vi "RT.vi"() -> ()   [LabVIEW 2020]
uses:
  <vilib>/FPGAPlugInAG/cRIO-9054/niLvFpga_Open_cRIO-9054.vi
  <vilib>/FPGAPlugInAG/cRIO-9054/niLvFpga_Reset_cRIO-9054.vi
  <vilib>/Utility/error.llb/Error Cluster From Error Code.vi
  <vilib>/rvi/errors/niLvFpgaAdjustHostInterfaceError.vi
  <vilib>/FPGAPlugInAG/cRIO-9054/niLvFpga_Run_cRIO-9054.vi
  <vilib>/FPGAPlugInAG/cRIO-9054/niLvFpga_Close_cRIO-9054.vi
  <vilib>/rvi/interface/nirviOpenFPGA/nirviOpenFPGA.xnode
  FPGA Bitfiles/8192.lvbitx
  <vilib>/rvi/interface/nirviMethod/nirviMethod.xnode
  <vilib>/rvi/interface/nirviReadWriteControl/nirviReadWriteControl.xnode
  <vilib>/rvi/interface/nirviCloseFPGA/nirviCloseFPGA.xnode
  <vilib>/rvi/errors/niLvFpgaMergeErrorWithErrorCode.vi
  <vilib>/FPGAPlugInAG/cRIO-9054/niLvFpga_ReadFifo_cRIO-9054.vi
  NiFpgaLv.dll
  <vilib>/FPGAPlugInAG/cRIO-9054/niLvFpga_StartFifo_cRIO-9054.vi
panel:
  in  "FFT length":i32=8192
  out "Timing Chart":waveform(i16)(graph)
  in  "FFT loop iterations":i32
  in  "auto stop":bool=TRUE
  out "FFT time (uSec)":u32
  out "data collection time (uSec)":u32
  out "FFT Spectrum":waveform(dbl)(graph)
  out "Actual loop rate (Hz)":dbl
  out "aquired data":waveform(dbl)(graph)
  in  "number of date points":i32=9000
  out "Timed Out?":bool
  in  "requested Loop rate (Hz)":u32=1000
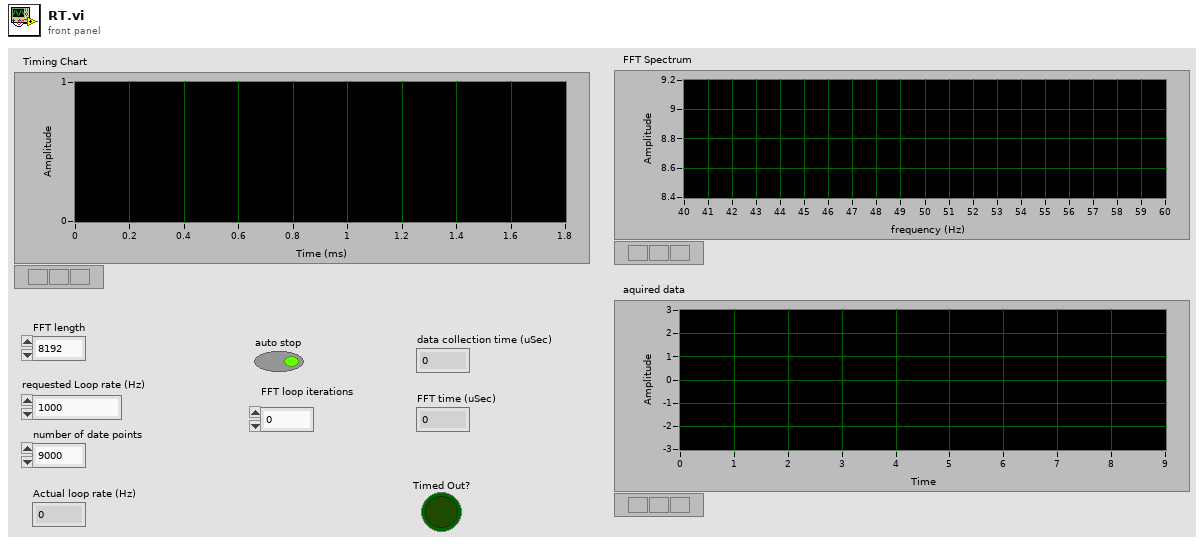
[diagram p1: front panel]
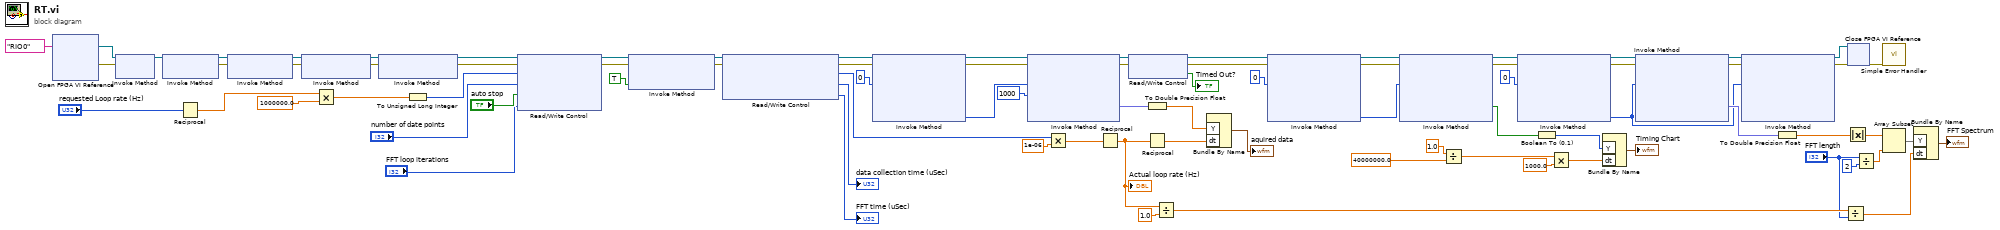
[diagram p0: block diagram]
diagram:
  n1 = xnode "Open FPGA VI Reference"("resource name"=tag "RIO0") -> ("FPGA VI Reference Out"=w33:refnum<k20>, "error out"=w32:errorcluster)  [unwired: 1 in]
  n2 = xnode "Invoke Method"("FPGA VI Reference In"=w33, "error in"=w32) -> ("FPGA VI Reference Out"=w11:refnum<k20>)  [unwired: 1 out]
  n3 = xnode "Invoke Method"("FPGA VI Reference In"=w11) -> ("FPGA VI Reference Out"=w10:refnum<k20>, "error out"=w9:errorcluster)  [unwired: 1 in]
  n4 = Reciprocal(x="requested Loop rate (Hz)") -> (1/x=w69:dbl)
  n5 = xnode "Invoke Method"("FPGA VI Reference In"=w10, "error in"=w9) -> ("FPGA VI Reference Out"=w15:refnum<k20>, "error out"=w14:errorcluster)
  n6 = xnode "Invoke Method"("FPGA VI Reference In"=w15, "error in"=w14) -> ("FPGA VI Reference Out"=w13:refnum<k20>, "error out"=w12:errorcluster)
  n7 = Multiply(x=w69, y=1000000.0) -> (x*y=w67:dbl)
  n8 = xnode "Invoke Method"("FPGA VI Reference In"=w13, "error in"=w12) -> ("FPGA VI Reference Out"=w18:refnum<k20>, "error out"=w17:errorcluster)
  n9 = To Unsigned Long Integer(number=w67) -> (unsigned 32bit integer=w66:u32)
  n10 = xnode "Read/Write Control"("FPGA VI Reference In"=w18, "error in"=w17, "Rate (uSec)"=w66, "Loop number"="number of date points", "auto stop"="auto stop", "FFT loop iterations"="FFT loop iterations") -> ("FPGA VI Reference Out"=w81:refnum<k20>, "error out"=w80:errorcluster)
  n11 = xnode "Invoke Method"("FPGA VI Reference In"=w81, "error in"=w80, "Wait Until Done (F)"=TRUE) -> ("FPGA VI Reference Out"=w77:refnum<k20>, "error out"=w76:errorcluster)
  n12 = xnode "Read/Write Control"("FPGA VI Reference In"=w77, "error in"=w76) -> ("FPGA VI Reference Out"=w30:refnum<k20>, "error out"=w29:errorcluster, "Actual loop rate"=w72:u32, "data collection time (uSec)"=→"data collection time (uSec)":u32, "FFT time (uSec)"=→"FFT time (uSec)":u32)
  n13 = xnode "Invoke Method"("FPGA VI Reference In"=w30, "error in"=w29, "Number of Elements"=u32 0) -> ("FPGA VI Reference Out"=w28:refnum<k20>, "error out"=w27:errorcluster, "Elements Remaining"=w25:u32)  [unwired: 1 in, 1 out]
  n14 = xnode "Invoke Method"("FPGA VI Reference In"=w28, "error in"=w27, "Number of Elements"=w25, "Timeout (ms)"=1000) -> ("FPGA VI Reference Out"=w75:refnum<k20>, "error out"=w74:errorcluster, "Data"=w39:fxp<+/-,24,7>[])  [unwired: 1 out]
  n15 = Multiply(x=w72, y=1e-06) -> (x*y=w70:dbl)
  n16 = Reciprocal(x=w70) -> (1/x=w35:dbl)
  "Actual loop rate (Hz)" <- w35
  n17 = xnode "Read/Write Control"("FPGA VI Reference In"=w75, "error in"=w74) -> ("FPGA VI Reference Out"=w46:refnum<k20>, "error out"=w45:errorcluster, "Timed Out?"=→"Timed Out?":bool)
  n18 = Reciprocal(x=w35) -> (1/x=w62:dbl)
  n19 = To Double Precision Float(number=w39) -> (double precision float=w63:dbl[])
  n20 = Divide(x=w35, y=1.0) -> (x/y=w54:dbl)
  n21 = Bundle By Name("Y"=w63, "dt"=w62) -> (→"aquired data":waveform(dbl))  [unwired: 1 in]
  n22 = xnode "Invoke Method"("FPGA VI Reference In"=w46, "error in"=w45, "Number of Elements"=u32 0) -> ("FPGA VI Reference Out"=w51:refnum<k20>, "error out"=w50:errorcluster, "Elements Remaining"=w49:u32)  [unwired: 1 in, 1 out]
  n23 = xnode "Invoke Method"("FPGA VI Reference In"=w51, "error in"=w50, "Number of Elements"=w49) -> ("FPGA VI Reference Out"=w44:refnum<k20>, "error out"=w43:errorcluster, "Data"=w48:bool[])  [unwired: 1 in, 1 out]
  n24 = Divide(x=1.0, y=40000000.0) -> (x/y=w3:dbl)
  n25 = xnode "Invoke Method"("FPGA VI Reference In"=w44, "error in"=w43, "Number of Elements"=u32 0) -> ("FPGA VI Reference Out"=w59:refnum<k20>, "error out"=w58:errorcluster, "Elements Remaining"=w19:u32)  [unwired: 1 in, 1 out]
  n26 = Boolean To (0,1)(Boolean=w48) -> (0, 1=w7:i16[])
  n27 = Multiply(x=w3, y=1000.0) -> (x*y=w2:dbl)
  n28 = Bundle By Name("Y"=w7, "dt"=w2) -> (→"Timing Chart":waveform(i16))  [unwired: 1 in]
  n29 = xnode "Invoke Method"("FPGA VI Reference In"=w59, "error in"=w58, "Number of Elements"=w19) -> ("FPGA VI Reference Out"=w64:refnum<k20>, "error out"=w61:errorcluster, "Data"=w24:fxp<+/-,32,21>[])  [unwired: 1 in, 1 out]
  n30 = xnode "Invoke Method"("FPGA VI Reference In"=w64, "error in"=w61, "Number of Elements"=w19) -> ("FPGA VI Reference Out"=w40:refnum<k20>, "error out"=w16:errorcluster)  [unwired: 1 in, 2 out]
  n31 = To Double Precision Float(number=w24) -> (double precision float=w34:dbl[])
  n32 = Divide(x=w54, y="FFT length") -> (x/y=w53:dbl)
  n33 = Absolute Value(x=w34) -> (abs(x)=w23:dbl[])
  n34 = xnode "Close FPGA VI Reference"("FPGA VI Reference In"=w40, "error in"=w16) -> ("error out"=w65:errorcluster)
  n35 = Divide(x="FFT length", y=2) -> (x/y=w41:dbl)
  n36 = call <vilib>:"Simple Error Handler.vi"("error in (no error)"=w65) -> ()  [unwired: 4 in, 5 out]
  n37 = Array Subset(array=w23, length=w41) -> (w20:dbl[])  [unwired: 1 in]
  n38 = Bundle By Name("Y"=w20, "dt"=w53) -> (→"FFT Spectrum":waveform(dbl))  [unwired: 1 in]
